vi "Measure.vi"(6 "timeout in ms (1000)":i32=1000, 8 "error in (no error)":errorcluster, 11 "MeasuringDevice":refnum<class "MeasuringDevice.lvclass">) -> (0 "error out":errorcluster, 2 "buffer":i32, 3 "MeasuringDevice out":refnum<class "MeasuringDevice.lvclass">)   [LabVIEW 2017, in "MeasuringDevice.lvclass"]
doc: "---------------------------------------------------------------\nJKI State Machine Objects™\nhttp://jki.net/state-machine-objects/\nCopyright (C) 2005-2015, JKI <info@jki.net>\nALL RIGHTS RESERVEDJKI State Machine Objects (SMO) 1.0.0.4\nJKI - JKI\nCopyright (c) 2015, JKI"
uses:
  MeasuringDevice.lvclass
  MeasuringDevice.lvclass/MeasuringDevice.ctl
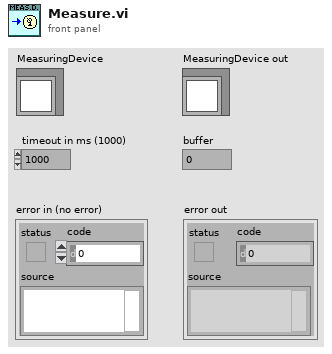
[diagram p1: front panel]
types:
  T1 = typedef "MeasuringDevice.lvclass/PrivateData--Ref.ctl" = refnum<data-value>
  T2 = typedef "MeasuringDevice.lvclass/PrivateData--Cluster.ctl" = cluster{"Configuration":T3, "Public Events":T4, "Protected Events":T5, "Data":string, "Dependencies":T6, "Private Events":T7}
  T3 = typedef "MeasuringDevice.lvclass/Configuration--Cluster.ctl" = cluster{"Suffix":string}
  T4 = typedef "MeasuringDevice.lvclass/PublicEvents--Cluster.ctl" = cluster{"Data Changed":refnum<user-event>, "MeasurementCompleted":refnum<user-event>}
  T5 = typedef "MeasuringDevice.lvclass/ProtectedEvents--Cluster.ctl" = cluster{"API_Template":refnum<user-event>}
  T6 = typedef "MeasuringDevice.lvclass/Dependencies--Cluster.ctl" = cluster{"CircularBuffer":refnum<class "CircularBuffer.lvclass">}
  T7 = typedef "MeasuringDevice.lvclass/PrivateEvents--Cluster.ctl" = cluster{"MakeMeasurement":refnum<user-event>}
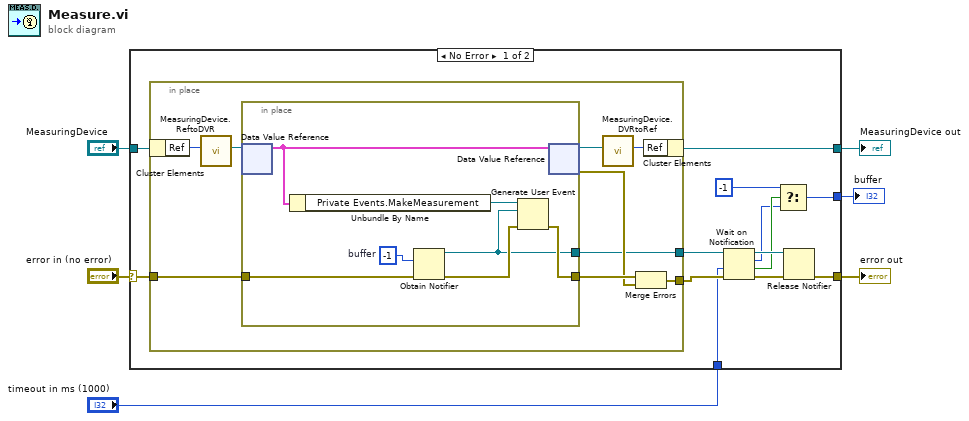
[diagram p0: block diagram]
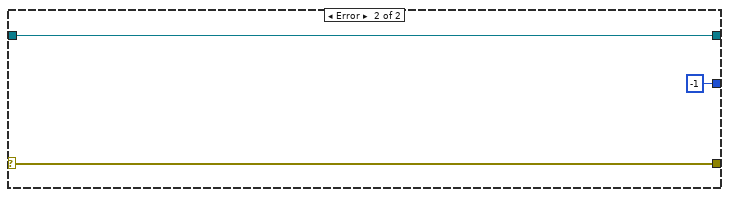
[diagram p2: hidden frame]
diagram:
  n1 = case shown="No Error" "error in (no error)" {
    selector: "error in (no error)" -> [w17 w38]
    tunnel: [w11 w38] -> w5
    tunnel: [w18 w37] -> w6
    tunnel: "MeasuringDevice" -> [w19 w37]
    tunnel: "timeout in ms (1000)" -> [w14 _]
    tunnel: [w7 -1 ("buffer")] -> w1
    frame No Error {
      n2 = in-place {
        in-place-border: w17 -> [w28]
        in-place-border: [w25] -> w15
        in-place-border: [w20] -> w16
        n3 = in-place-cluster #1(w19) -> ("Ref"=w24:u32)
        n4 = call "MeasuringDevice.ReftoDVR.vi"("Ref"=w24) -> ("Ref"=w22:T1)  [unwired: 10 in]
        n5 = in-place {
          in-place-border: w28 -> [w31]
          in-place-border: [w33] -> w27
          in-place-border: [w29] -> w20
          w32 = -1  # buffer
          n6 = in-place-dvr #2(w22) -> (w35:T2)  [unwired: 1 out]
          n7 = Unbundle By Name(w35) -> ("Private Events.MakeMeasurement"=w34:refnum<user-event>)
          n8 = Obtain Notifier(notification data type=w32, error in (no error)=w31) -> (notifier out=w29:refnum<notifier>, error out=w30:errorcluster)  [unwired: 2 in, 1 out]
          n9 = Generate User Event(user event=w34, event data cluster=w29, error in=w30) -> (error out=w33:errorcluster)  [unwired: 1 in, 1 out]
          n10 = in-place-dvr #2(w35) -> (w23:T1, w26:errorcluster)
        }
        n11 = call "MeasuringDevice.DVRtoRef.vi"("Ref"=w23) -> ("Ref"=w21:u32)  [unwired: 10 in]
        n12 = Merge Errors(w27, w26) -> (w25:errorcluster)
        n13 = in-place-cluster #1("Ref"=w21) -> (w18:refnum<class "MeasuringDevice.lvclass">)
      }
      n14 = Wait on Notification(notifier=w16, timeout in ms (-1)=w14, error in (no error)=w15) -> (notifier out=w12:refnum<notifier>, notification=w8:i32, timed out?=w10:bool, error out=w13:errorcluster)  [unwired: 1 in]
      n15 = Select(t=-1, s=w10, f=w8) -> (s? t:f=w7:i32)
      n16 = Release Notifier(notifier=w12, error in (no error)=w13) -> (error out=w11:errorcluster)  [unwired: 1 in, 2 out]
    }
    frame Error {
    }
  }
  "error out" <- w5
  "MeasuringDevice out" <- w6
  "buffer" <- w1
